vi "cm_Level Color Popup.vi"() -> ()   [LabVIEW 2009, in "Channel Monitor.xctl"]
uses:
  Channel Monitor.xctl
  <vilib>/Utility/error.llb/DialogType.ctl
panel:
  out "error out":errorcluster
  in  "Done":bool
  in  "Peak":u32(colorbox)=16711680
  in  "Current":u32(colorbox)=6618880
  # "Current"
  # "Peak"
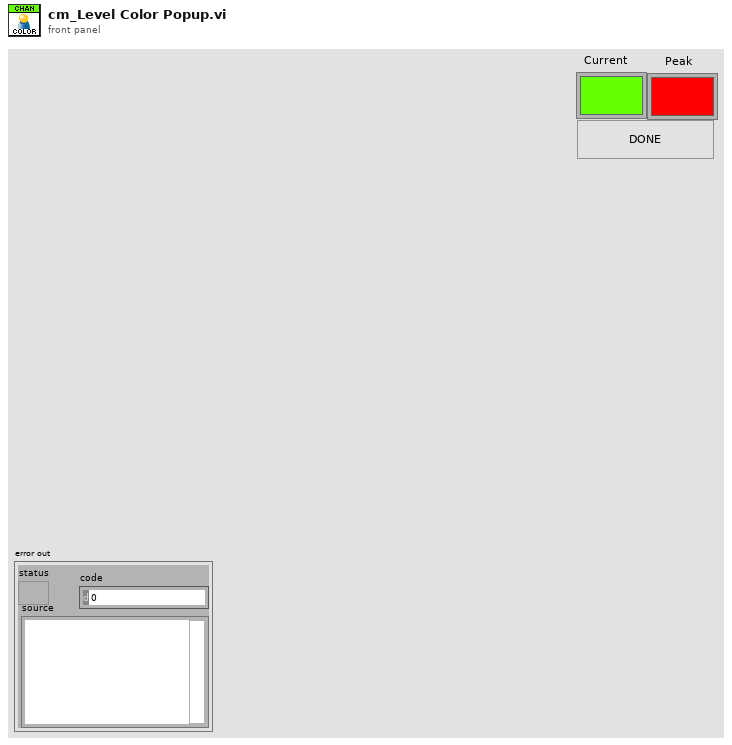
[diagram p1: front panel]
types:
  T1 = typedef "amc_Message Queue.ctl" = refnum<queue>
  T2 = typedef "DialogType.ctl" = u16
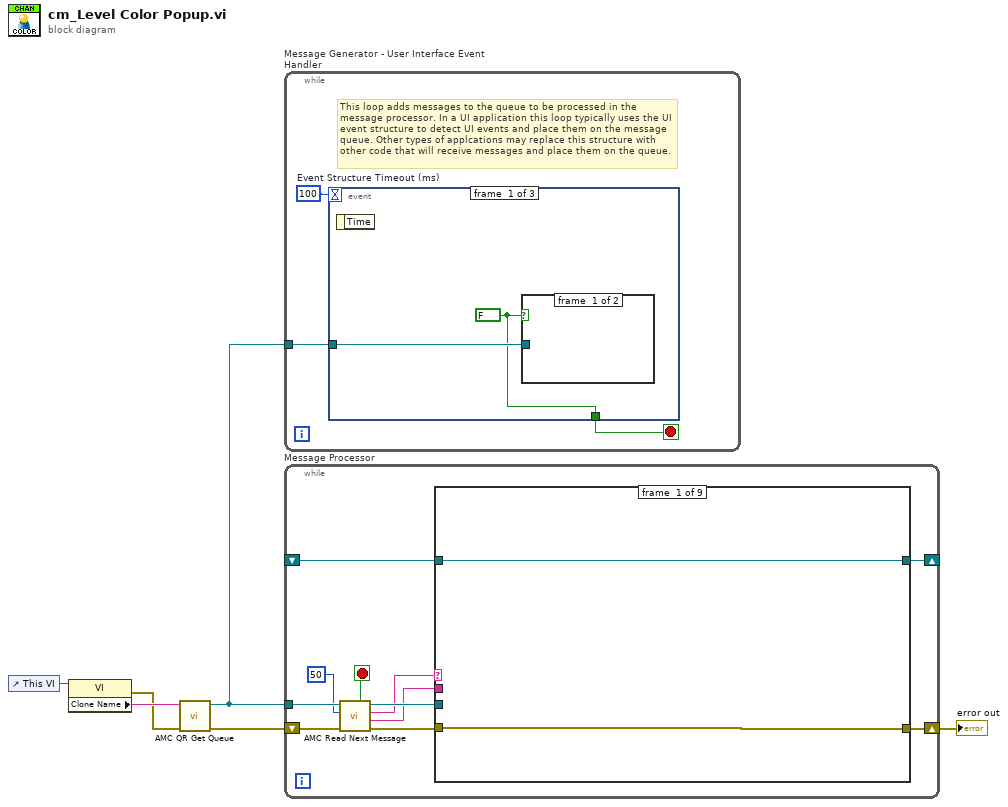
[diagram p0: block diagram]
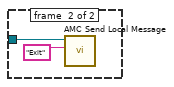
[diagram p2: hidden frame]
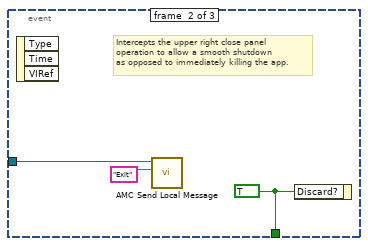
[diagram p3: hidden frame]
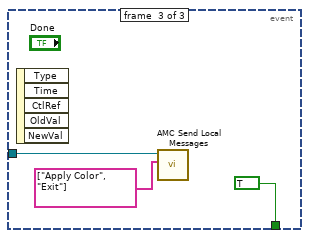
[diagram p4: hidden frame]
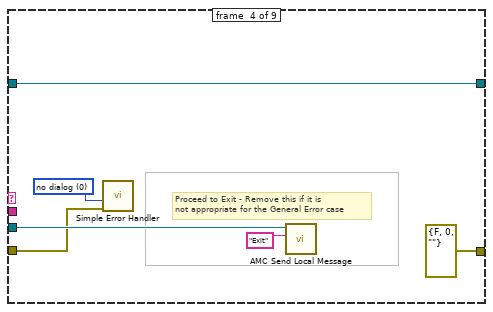
[diagram p7: hidden frame]
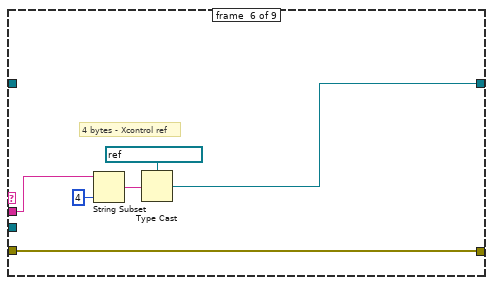
[diagram p9: hidden frame]
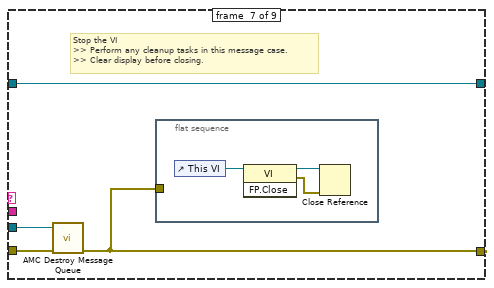
[diagram p10: hidden frame]
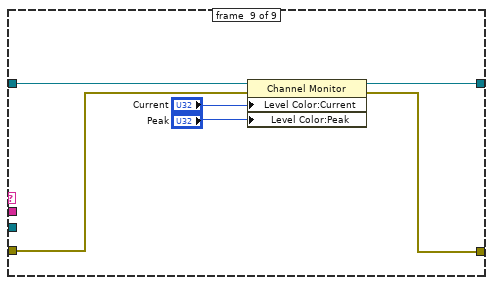
[diagram p12: hidden frame]
diagram:
  n1 = control-ref of="This VI"() -> (w4:refnum<vi>)
  n2 = property class="VI"(reference=w4) -> (error out=w1:errorcluster, "Clone Name"=w5:string)  [unwired: 1 in, 1 out]
  n3 = call <userlib>:"AMC QR Get Queue .vi"("error in (no error)"=w1, "Name"=w5) -> ("error out"=w2:errorcluster, "Queue Out"=w6:T1)  [unwired: 8 in]
  n4 = while "Message Generator - User Interface Event Handler" {
    tunnel: w6 -> [w7]
    stop <- w8 stop-if-true
    w9 = 100  # Event Structure Timeout (ms)
    # "This loop adds messages to the queue to be processed in the message processor. In a UI application this loop typically uses the UI event structure to detect UI events and place them on the message queue. Other types of applcations may replace this structure with other code that will receive messages and place them on the queue."
    n5 = event shown="[2] \"Done\": Value Change" {
      selector: _ -> [_ _ _]
      dyn-events: _ -> [_ _ _]
      timeout: w9 -> [_ _ _]
      tunnel: [w10 w16 TRUE ("Discard?")] -> w8
      tunnel: w7 -> [w11 w15 w18]
      event #0 {
        w10 = FALSE
        n6 = event-data() -> ()  [unwired: 2 out]
        n7 = case shown="True" w10 {
          tunnel: w11 -> [_ w12]
          frame #0 {
          }
          frame #1 {
            n8 = call <userlib>:"AMC Send Local Message.vi"("Message Name"="Exit", "Message Queue in"=w12) -> ()  [unwired: 4 in, 6 out]
          }
        }
      }
      event #1 {
        w16 = TRUE ("Discard?")
        # "Intercepts the upper right close panel\noperation to allow a smooth shutdown\nas opposed to immediately killing the app."
        n9 = event-data() -> ()  [unwired: 4 out]
        n10 = call <userlib>:"AMC Send Local Message.vi"("Message Name"="Exit", "Message Queue in"=w15) -> ()  [unwired: 4 in, 6 out]
        n11 = event-data("Discard?"=w16) -> ()  [unwired: 1 in, 1 out]
      }
      event #2 {
        n12 = event-data() -> ()  [unwired: 6 out]
        n13 = call <userlib>:"AMC Send Local Messages.vi"("Message Names"=string[] ["Apply Color", "Exit"], "Message Queue in"=w18) -> ()  [unwired: 8 in, 2 out]
      }
    }
  }
  n14 = while "Message Processor" {
    shift-left: w2 -> [w29]
    shift-right: [w30] -> w3
    tunnel: w6 -> [w26]
    shift-right: [w21] -> _
    shift-left: _ -> [w20]
    stop <- w25 stop-if-true
    n15 = call <userlib>:"AMC Read Next Message.vi"("error in (no error)"=w29, "timeout (1ms)"=50, "Message Queue in"=w26) -> ("error out"=w28:errorcluster, "Message Value"=w23:string, "Message Name"=w24:string, "Message Queue out"=w27:T1, "Exit Process"=w25:bool)  [unwired: 1 in, 3 out]
    n16 = case shown="\"Initialize\"" w24 {
      tunnel: w23 -> [_ _ _ _ _ w47 _ _ _]
      tunnel: w28 -> [w32 w34 w36 w39 w44 w46 w53 w59 w63]
      tunnel: [w32 w34 w36 errorcluster {"status"=FALSE, "code"=0, "source"=""} ("error out") w44 w46 w52 w59 w62] -> w30
      tunnel: w27 -> [_ _ _ w41 _ _ w54 _ _]
      tunnel: [w31 w33 w35 w37 w43 w45 w51 w58 w60] -> w21
      tunnel: w20 -> [w31 w33 w35 w37 w43 _ w51 w58 w61]
      frame #0 {
        # "Dummy case to add a seperator in the Case Structure menu"
      }
      frame #1 {
      }
      frame #2 {
        # "Call this case if a message is received that is not handled \nby any other case. Typically this is a programming error\nas a result of a typo or unhandled message/missing message handler."
      }
      frame #3 {
        w40 = T2 0 items=["no dialog", "OK message", "continue or stop message", "OK message + warnings", "continue/stop + warnings"] ("type of dialog (OK msg:1)")
        # "Proceed to Exit - Remove this if it is\nnot appropriate for the General Error case"
        # "General Error Case - this case is called if an error is passed using the error cluster below. Typically most new errors should be handed in each individual case and not passed in the rror cluster. If necessary a custom error handler case should be added and called from other cases."
        n17 = call <vilib>:"Simple Error Handler.vi"("type of dialog (OK msg:1)"=w40, "error in (no error)"=w39) -> ()  [unwired: 8 out]
        n18 = call <userlib>:"AMC Send Local Message.vi"("Message Name"="Exit", "Message Queue in"=w41) -> ()  [unwired: 4 in, 6 out]
      }
      frame #4 {
        # "Dummy case to add a seperator in the Case Structure menu"
      }
      frame #5 {
        # "4 bytes - Xcontrol ref"
        # "Initialize the state variables and user interface"
        n19 = String Subset(string=w47, length (rest)=4 ("length (rest)")) -> (substring=w49:string)  [unwired: 1 in]
        n20 = Type Cast(type=refnum<vi> refnum ("Channel Monitor"), x=w49) -> (*(type *) &x=w45:refnum<vi>)
      }
      frame #6 {
        # "Stop the VI\n>> Perform any cleanup tasks in this message case.\n>> Clear display before closing."
        n21 = call <userlib>:"AMC Destroy Message Queue.vi"("error in (no error)"=w53, "Message Queue in"=w54) -> ("error out"=w52:errorcluster)  [unwired: 9 out]
        n22 = flat-sequence {
          tunnel: w52 -> [_]
          frame #0 {
            n23 = control-ref of="This VI"() -> (w55:refnum<vi>)
            n24 = invoke class="VI" method="FP.Close"(reference=w55) -> (reference out=w57:refnum<vi>, error out=w56:errorcluster)  [unwired: 2 in, 1 out]
            n25 = Close Reference(reference=w57, error in (no error)=w56) -> ()  [unwired: 1 out]
          }
        }
      }
      frame #7 {
        # "Dummy case to add a seperator in the Case Structure menu"
      }
      frame #8 {
        # "Dummy case to add a seperator in the Case Structure menu"
        n26 = property class="Channel Monitor"(reference=w61, error in=w63, "Level Color:Current"="Current", "Level Color:Peak"="Peak") -> (reference out=w60:refnum<vi>, error out=w62:errorcluster)
      }
    }
  }
  "error out" <- w3
